vi "PH_BlackBox.evt stop move.vi"(0 "i ref in":refnum<vi>, 2 "Instance":string="N/A", 5 "error in (no error)":errorcluster) -> (14 "i ref out":refnum<vi>, 19 "error out":errorcluster)   [LabVIEW 2014, in "PH_BlackBox.lvlib"]
doc: "This VI sends a stop command"
uses:
  PH_BlackBox.lvlib
  CS_Core/CSSystem/CoreLib/CoreLib.short 2 byte array.vi
  CS_Core/CSSystem/CoreLib/CoreLib.lvlib
  CS_Core/BaseProcess/BaseProcess.lvlib
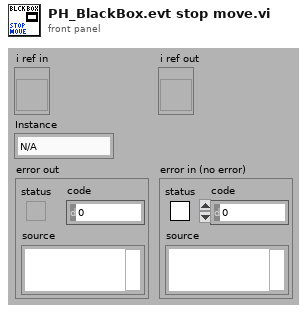
[diagram p1: front panel]
types:
  T1 = typedef "CoreDefs.rawDataType.ctl" = i8[]
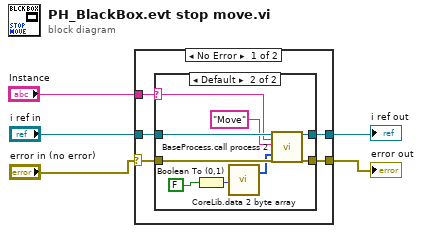
[diagram p0: block diagram]
diagram:
  n1 = case shown="No Error" "error in (no error)" {
    selector: "error in (no error)" -> [w6 w22]
    tunnel: [w10 w23] -> w1
    tunnel: [w9 w22] -> w2
    tunnel: "i ref in" -> [w8 w23]
    tunnel: "Instance" -> [w7 _]
    frame No Error {
      n2 = case shown="Default" w7 {
        selector: w7 -> [_ w13]
        tunnel: [w12 w21] -> w10
        tunnel: [w11 w20] -> w9
        tunnel: w8 -> [w12 w19]
        tunnel: w6 -> [w11 w18]
        frame "N/A" {
        }
        frame Default {
          n3 = Boolean To (0,1)(Boolean=FALSE) -> (0, 1=w16:i16)
          n4 = call-poly "CoreLib.data 2 byte array.vi"("i16"=w16) -> ("byteArray out"=w14:T1)  [unwired: 18 in]
          n5 = call "BaseProcess.call process 2.vi"("i ref in"=w19, "Object"=w13, "Selector"="Move", "Data"=w14, "error in (no error)"=w18) -> ("i ref out"=w21:refnum<vi>, "error out"=w20:errorcluster)  [unwired: 13 in]
        }
      }
    }
    frame Error {
    }
  }
  "error out" <- w2
  "i ref out" <- w1
